vi "ep_Motor Information.vi"(8 "error in (no error)":errorcluster, 10 "motor information":T1, 11 "nominal frequency":enum16{"50 Hz", "60 Hz"}(ring)) -> (0 "error out":errorcluster, 3 "information":T2)   [LabVIEW 2014, in "NI_EP_Motor Monitoring.lvlib"]
uses:
  <vilib>/addons/Electrical Power/Motor Monitoring/NI_EP_Motor Monitoring.lvlib
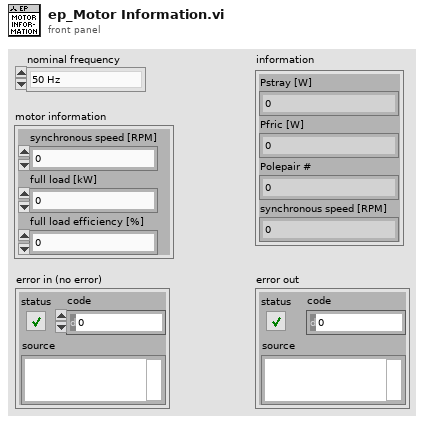
[diagram p1: front panel]
types:
  T1 = cluster{"synchronous speed [RPM]":dbl, "full load [kW]":dbl, "full load efficiency [%]":dbl}
  T2 = cluster{"Pstray [W]":dbl, "Pfric [W]":dbl, "Polepair #":i32, "synchronous speed [RPM]":dbl}
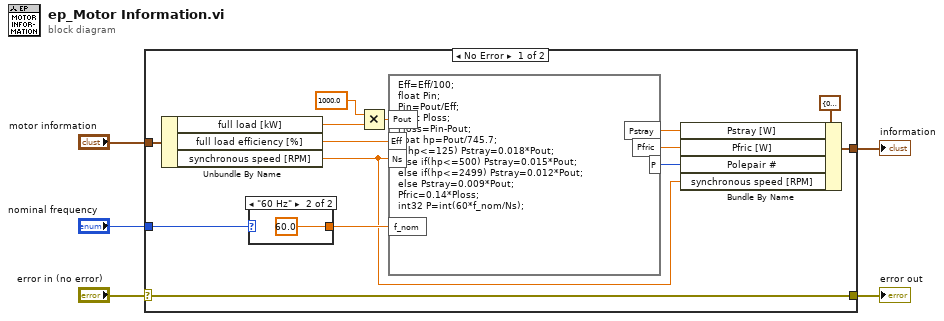
[diagram p0: block diagram]
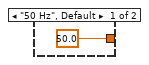
[diagram p2: hidden frame]
diagram:
  n1 = case shown="No Error" "error in (no error)" {
    selector: "error in (no error)" -> [w13 w22]
    tunnel: "motor information" -> [w17 _]
    tunnel: "nominal frequency" -> [w15 _]
    tunnel: [w13 w22] -> w2
    tunnel: [w12 _] -> w1
    frame No Error {
      n2 = Unbundle By Name(w17) -> ("full load [kW]"=w7:dbl, "full load efficiency [%]"=w16:dbl, "synchronous speed [RPM]"=w9:dbl)
      n3 = case shown="\"60 Hz\"" w15 {
        tunnel: [50.0 60.0] -> w14
        frame "50 Hz", Default {
        }
        frame "60 Hz" {
        }
      }
      n4 = Multiply(x=1000.0, y=w7) -> (x*y=w8:dbl)
      n5 = formula code="Eff=Eff/100;\nfloat Pin;\nPin=Pout/Eff;\nfloat Ploss;\nPloss=Pin-Pout;\nfloat hp=Pout/745.7;\nif(hp<=125) Pstray=0.018*Pout;\nelse if(hp<=500) Pstray=0.015*Pout;\nelse if(hp<=2499) Pstray=0.012*Pout;\nelse Pstray=0.009*Pout;\nPfric=0.14*Ploss;\nint32 P=int(60*f_nom/Ns);"("Pout"=w8, "Eff"=w16, "Ns"=w9, "f_nom"=w14) -> ("Pstray"=w19:dbl, "Pfric"=w18:dbl, "P"=w11:i32)
      n6 = Bundle By Name(cluster=T2 {"Pstray [W]"=0.0, "Pfric [W]"=0.0, "Polepair #"=0, "synchronous speed [RPM]"=0.0} ("information"), "Pstray [W]"=w19, "Pfric [W]"=w18, "Polepair #"=w11, "synchronous speed [RPM]"=w9) -> (w12:T2)
    }
    frame Error {
    }
  }
  "information" <- w1
  "error out" <- w2
